vi "Example_OE1022 Sample.vi"() -> ()   [LabVIEW 2011]
uses:
  <vilib>/Utility/file.llb/Write To Spreadsheet File (DBL).vi
panel:
  out "输出数组":sgl[](array[numeric])
  out "diff_value":i32
  in  "Buffer":u16(ring) items=["R", "X", "Y", "Theta", "Rh1", "Xh1", "Yh1", "Theta h1", "Rh2", "Xh2", "Yh2", "Theta h2", "Noise", "A1", "A2", "A3", "A4", "E1", "E2", "E3", "E4", "Freq"]
  in  "Channel":i32(ring)=1 items=["1"=1, "2"=2, "3"=3, "4"=4]
  out "point":i32
  out "dis_flag":i32
  out "now_point":i32
  in  "Save Path":path=path "C:/Users/Joean/Desktop/123.xls"
  out "Output":sgl[](array[numeric])
  out "chart":sgl[](graph)
  in  "stop":bool
  in  "save":bool
  out "now_point":string
  out "Read Buffer":string
  in  "command":string
  in  "Remote Mode":u16(ring)=1 items=["USB", "RS232", "GPIB", "Ethernet"]
  in  "VISA resource name":refnum<visa-resource-name>
  in  "control_state":T1(ring)
  in  "drive_control":T2(ring)
  # "Tel          :   +86-020-84133345\nWebsite  :   www.ssi-instrument.com\nE-mail     :   support@si-instrument.com"
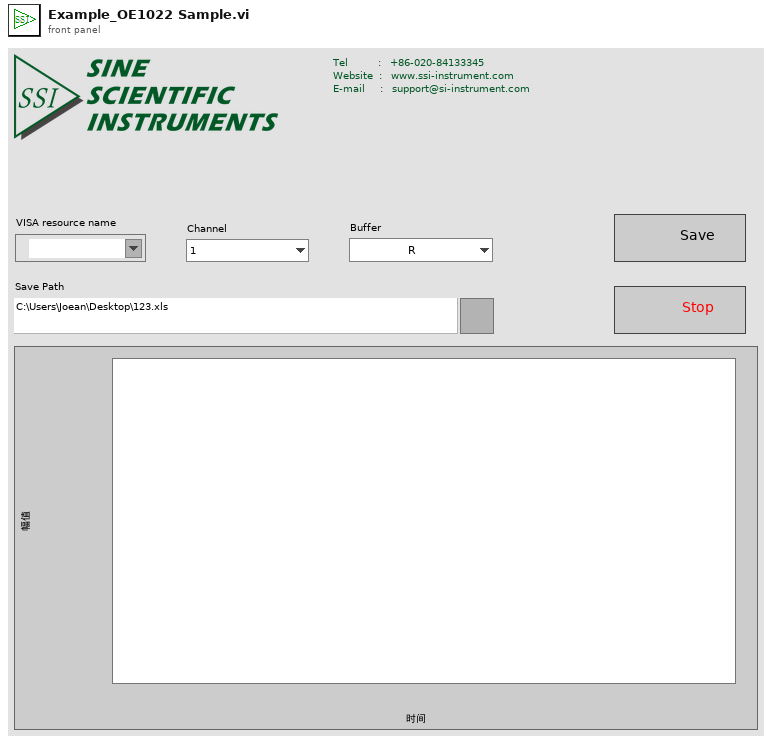
[diagram p1: front panel]
types:
  T1 = enum16{"connect", "initial", "idle", "set_channel", "sample", "save", "stop"}
  T2 = enum16{"idle", "initial", "write_cmd", "get_point", "read_data", "close"}
  T3 = enum16{"connect", "initial", "idle", "set_channel", "sample", "save", "stop", "close"}
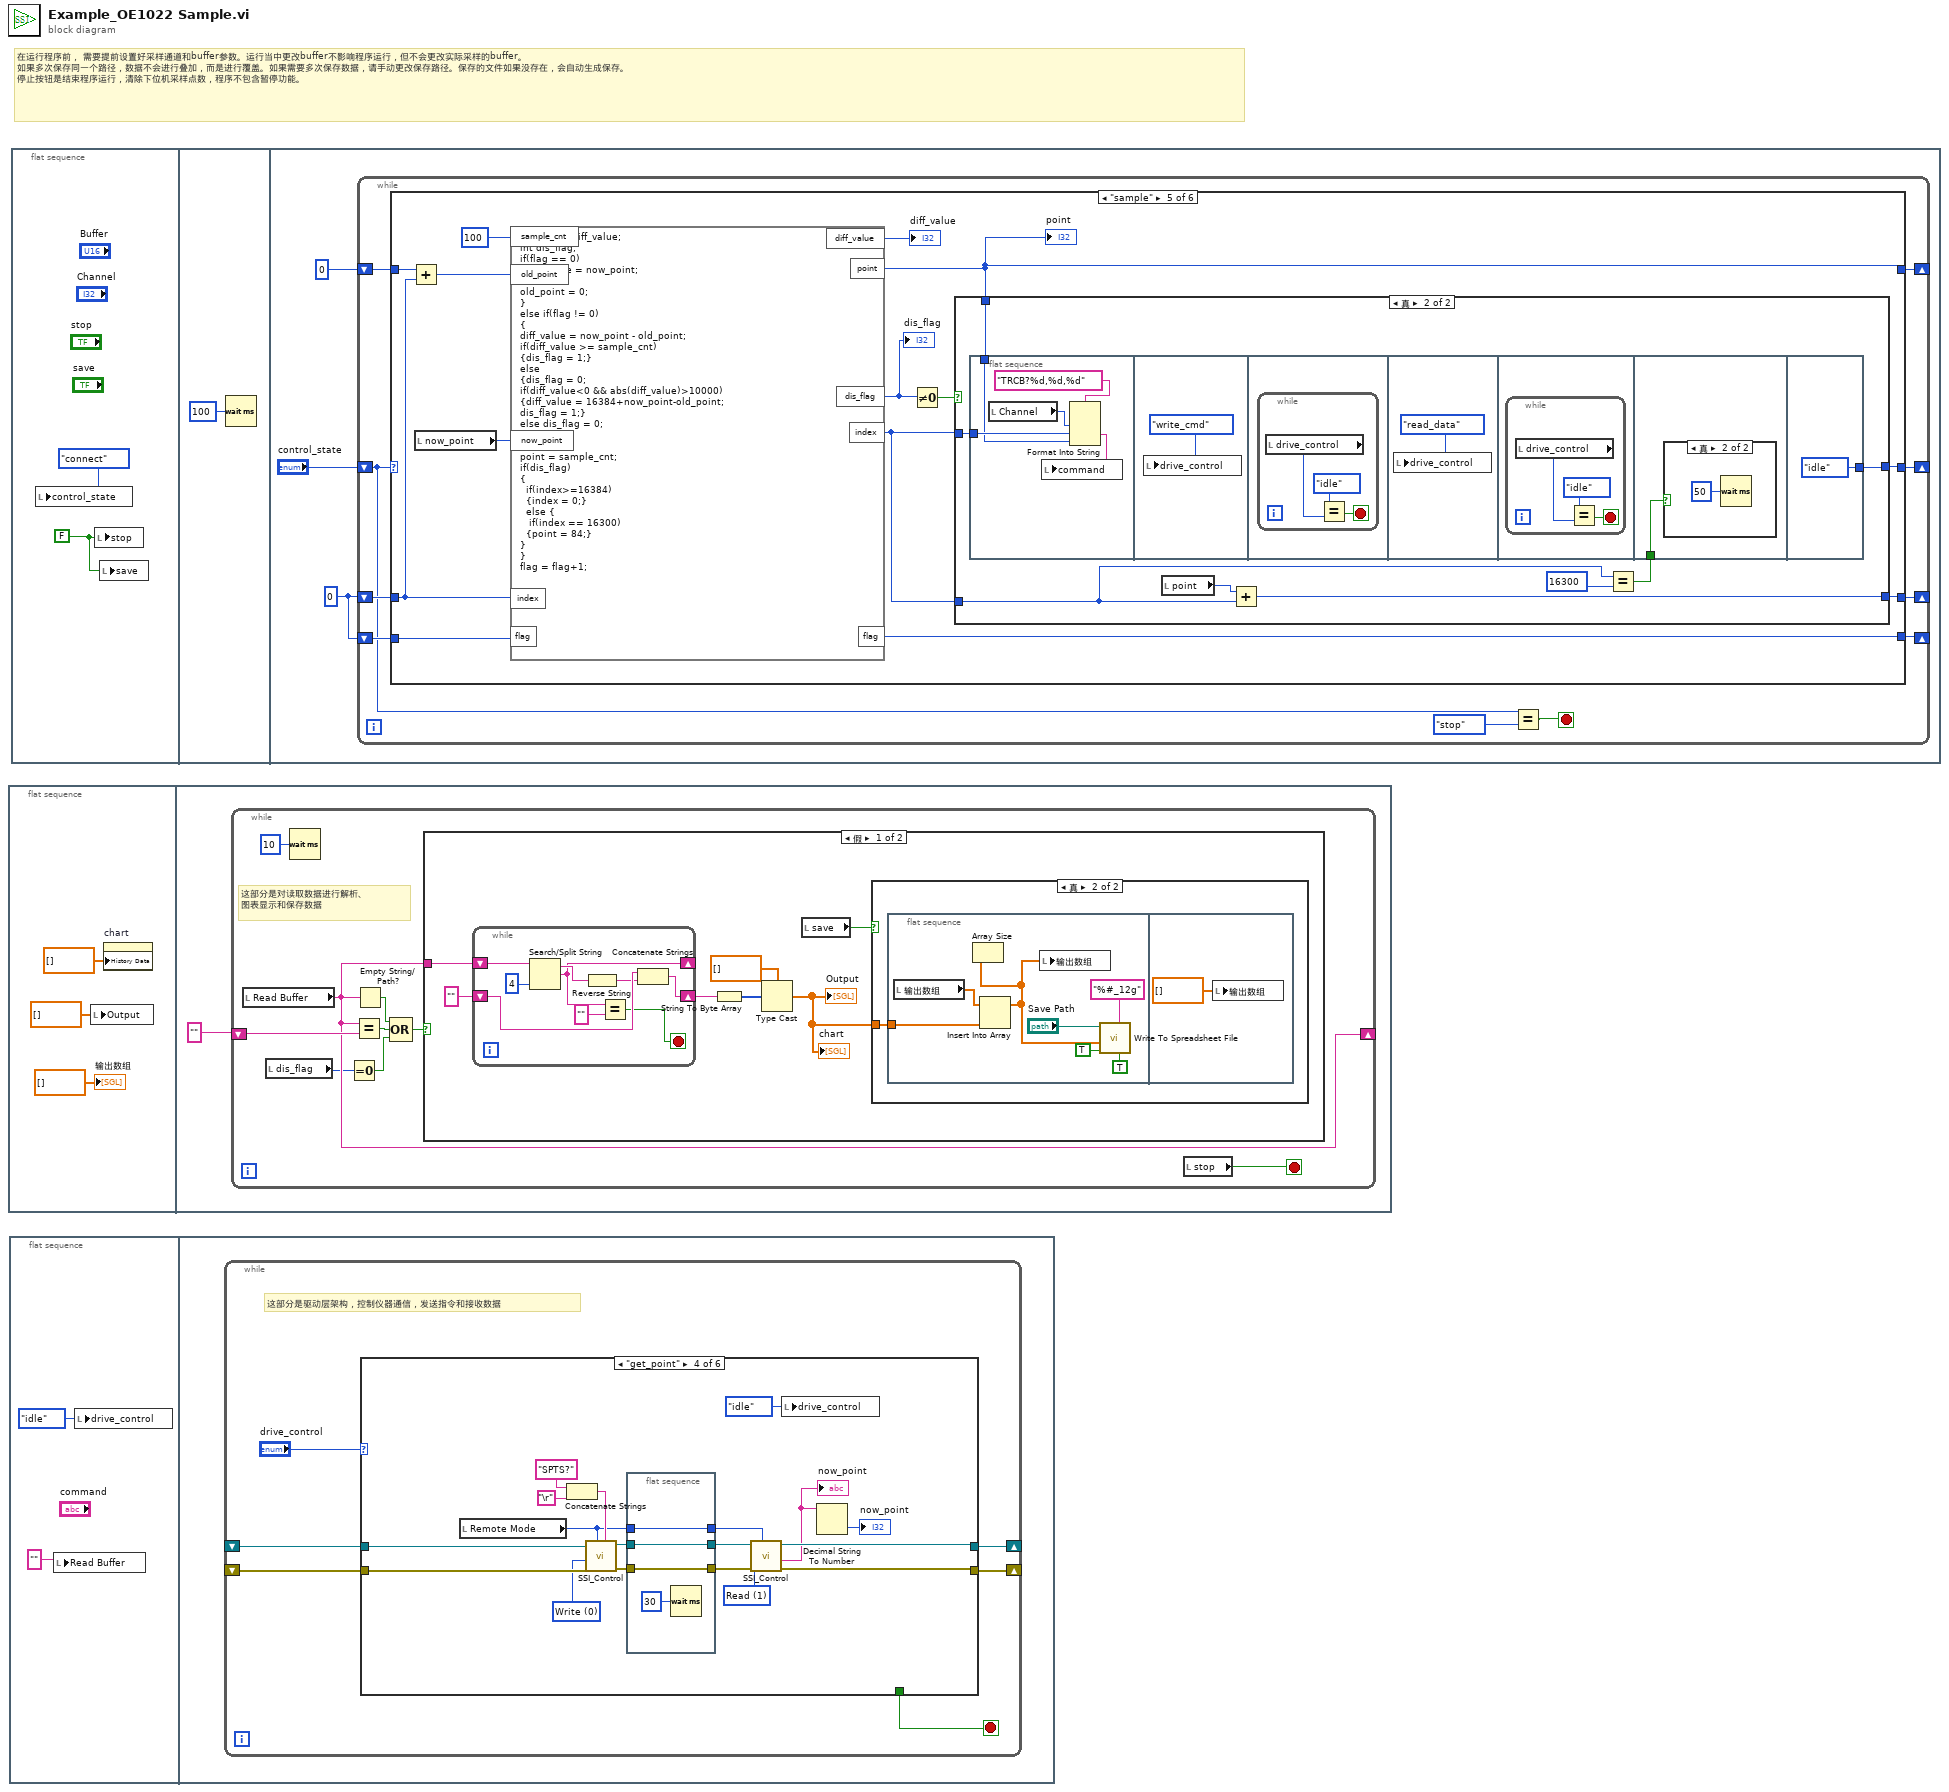
[diagram p0: block diagram]
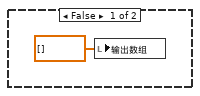
[diagram p2: hidden frame]
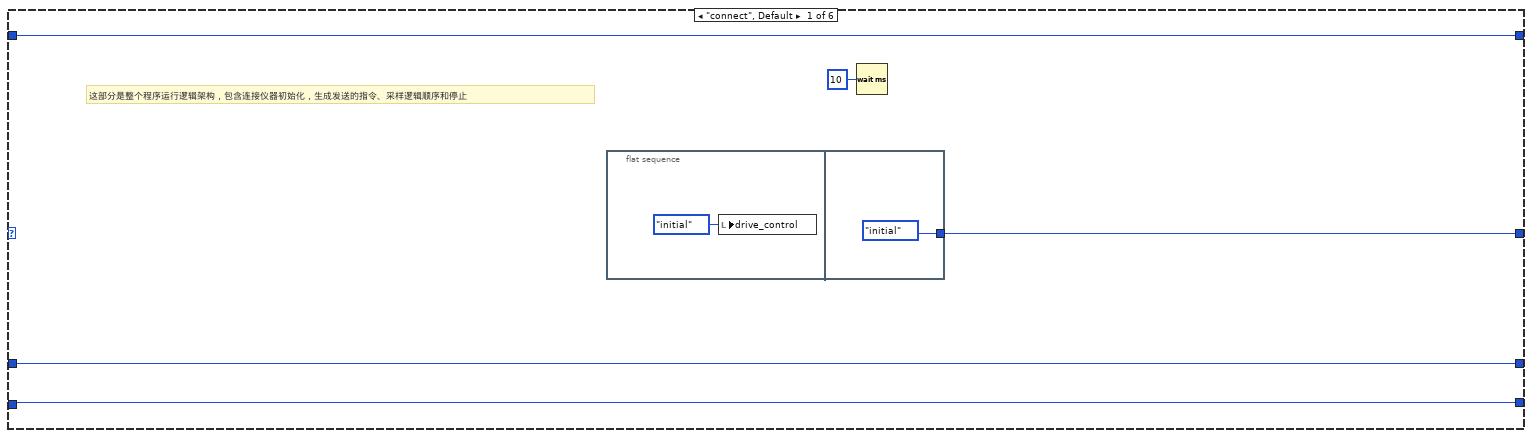
[diagram p4: hidden frame]
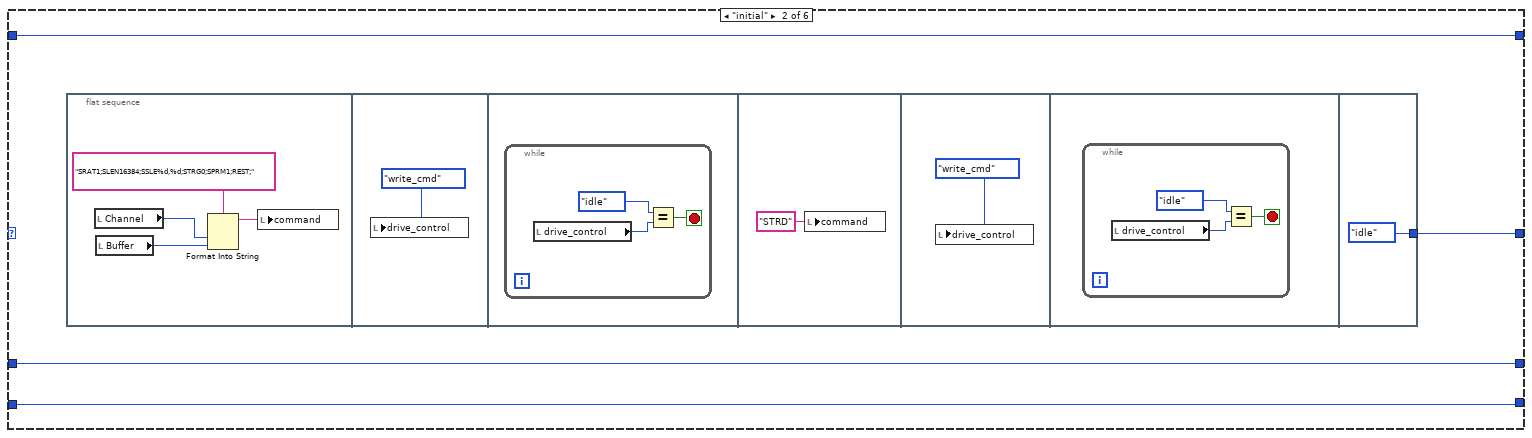
[diagram p5: hidden frame]
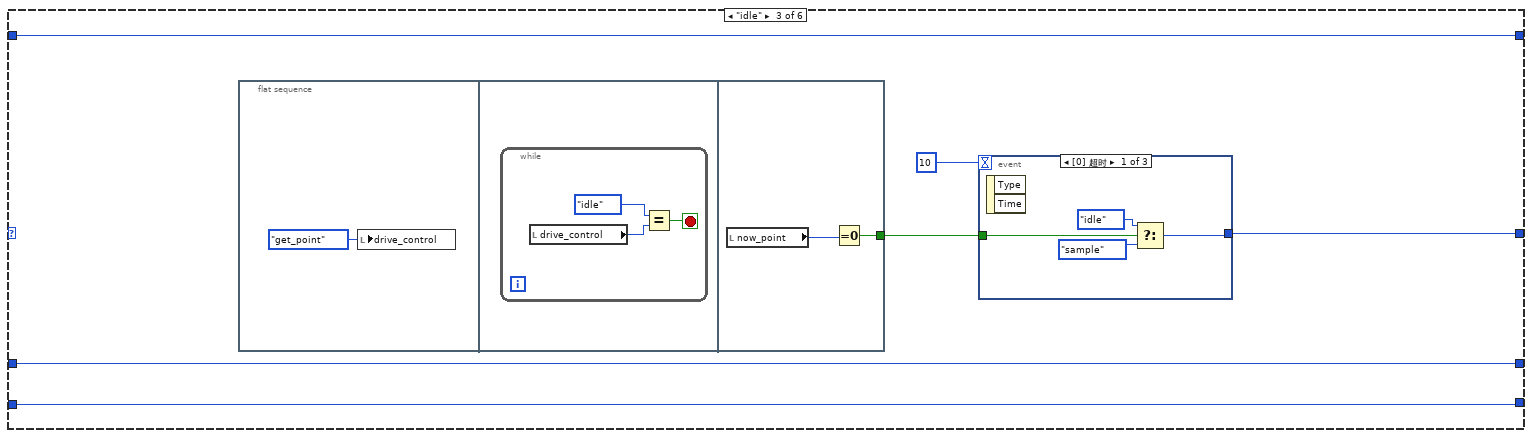
[diagram p6: hidden frame]
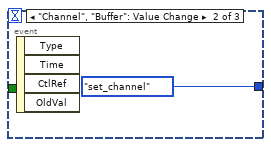
[diagram p7: hidden frame]
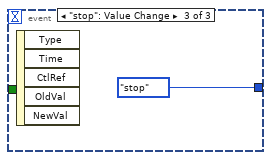
[diagram p8: hidden frame]
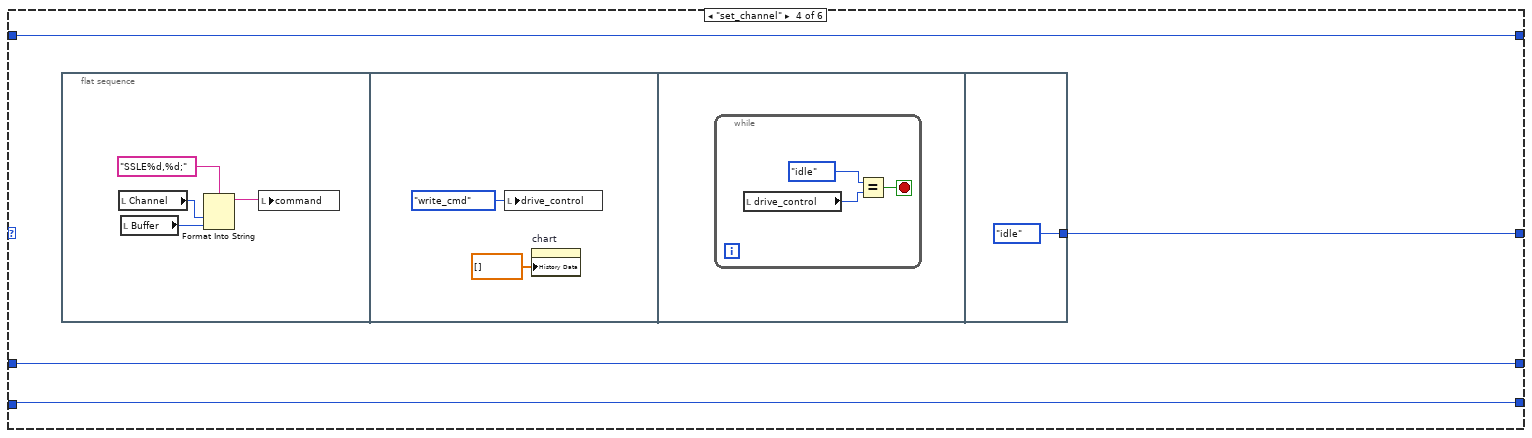
[diagram p9: hidden frame]
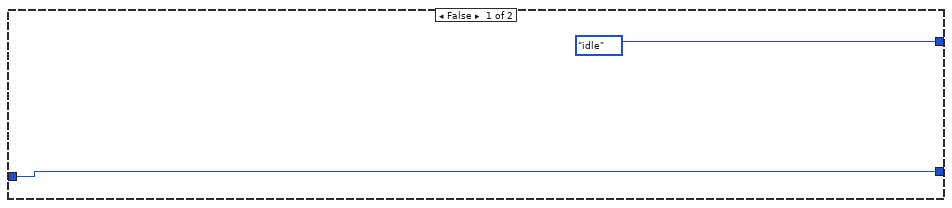
[diagram p10: hidden frame]
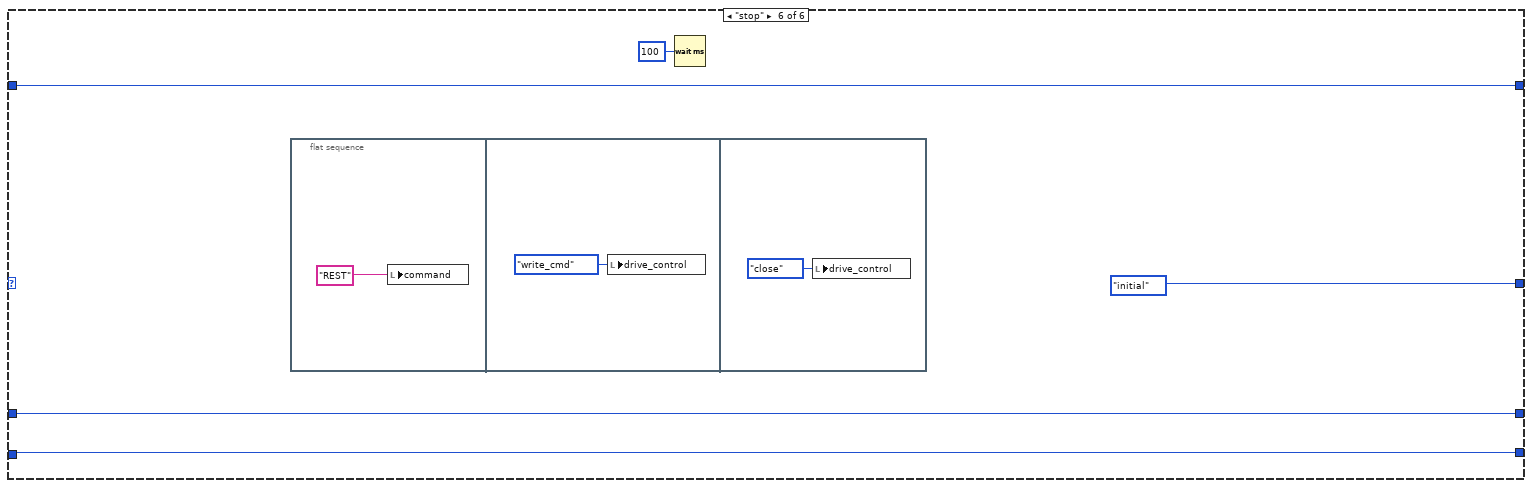
[diagram p12: hidden frame]
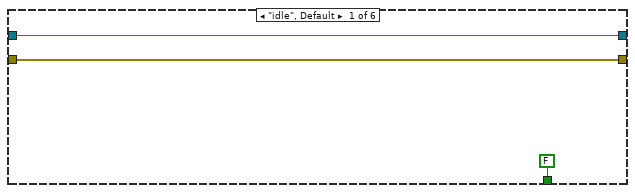
[diagram p13: hidden frame]
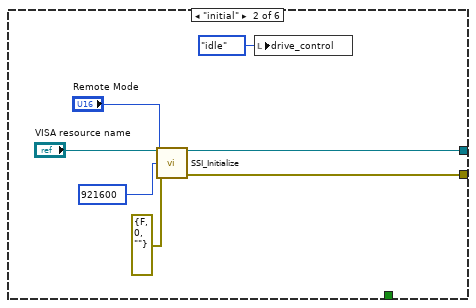
[diagram p14: hidden frame]
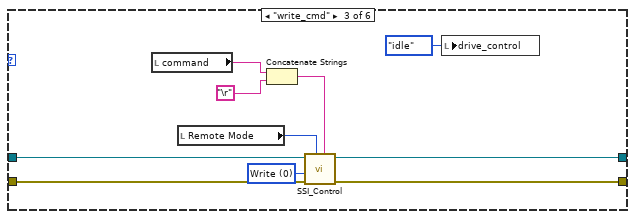
[diagram p15: hidden frame]
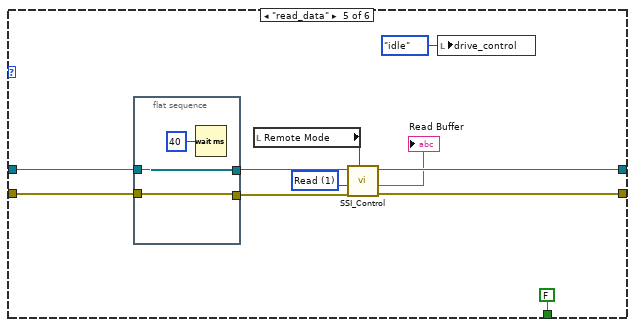
[diagram p16: hidden frame]
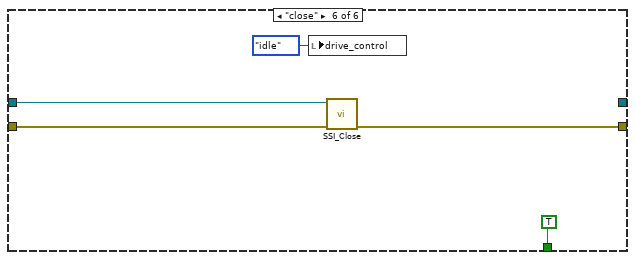
[diagram p17: hidden frame]
diagram:
  # "在运行程序前， 需要提前设置好采样通道和buffer参数。运行当中更改buffer不影响程序运行，但不会更改实际采样的buffer。\n如果多次保存同一个路径，数据不会进行叠加，而是进行覆盖。如果需要多次保存数据，请手动更改保存路径。保存的文件如果没存在，会自动生成保存。\n停止按钮是结束程序运行，清除下位机采样点数，程序不包含暂停功能。"
  n1 = flat-sequence {
    frame #0 {
      n2 = local write "Output"(sgl[] [] ("Output")) -> ()
      n3 = property on="chart" class="WFChart (严格)"("History Data"=sgl[] [] ("历史数据")) -> ()  [unwired: 2 in, 2 out]
      "输出数组" <- sgl[] [] ("输出数组")
    }
    frame #1 {
      n4 = while {
        shift-right: [w9] -> _
        shift-left: "" -> [w10]
        stop <- w12 stop-if-true
        # "这部分是对读取数据进行解析、\n图表显示和保存数据"
        n5 = local read "Read Buffer"() -> (w9:string)
        n6 = local read "dis_flag"() -> (w7:i32)
        n7 = Wait (ms)(milliseconds to wait=u32 10 ("等待时间（毫秒）")) -> ()  [unwired: 1 out]
        n8 = Equal To 0?(x=w7) -> (x = 0?=w6:bool)
        n9 = Equal?(x=w9, y=w10) -> (x = y?=w11:bool)
        n10 = Empty String/Path?(string/path=w9) -> (empty?=w8:bool)
        n11 = Compound Arithmetic op=OR(w8, w11, w6) -> (w5:bool)
        n12 = case shown="假" w5 {
          tunnel: w9 -> [w20 _]
          frame False {
            n13 = while {
              shift-right: [w33] -> _
              shift-left: w20 -> [w37]
              shift-right: [w34] -> w16
              shift-left: "" -> [w36]
              stop <- w31 stop-if-true
              n14 = Search/Split String(string=w37, offset (0)=4 ("偏移量(0)")) -> (substring before match=w38:string, match + rest of string=w33:string)  [unwired: 1 in, 1 out]
              n15 = Reverse String(1:w38) -> (0:w35:string)
              n16 = Equal?(x=w33, y="") -> (x = y?=w31:bool)
              n17 = Concatenate Strings(w36, w35) -> (w34:string)
            }
            n18 = String To Byte Array(string=w16) -> (unsigned byte array=w19:u8[])
            n19 = Type Cast(type=sgl[] [], x=w19) -> (*(type *) &x=w14:sgl[])
            "Output" <- w14
            "chart" <- w14
            n20 = local read "save"() -> (w15:bool)
            n21 = case shown="真" w15 {
              tunnel: w14 -> [_ w22]
              frame False {
                n22 = local write "输出数组"(sgl[] [] ("输出数组")) -> ()
              }
              frame True {
                n23 = flat-sequence {
                  tunnel: w22 -> [w25]
                  frame #0 {
                    n24 = local read "输出数组"() -> (w24:sgl[])
                    n25 = Insert Into Array(array=w24, new element=w25) -> (w23:sgl[])  [unwired: 1 in]
                    n26 = Array Size(array=w23) -> ()  [unwired: 1 out]
                    n27 = local write "输出数组"(w23) -> ()
                    n28 = call-poly <vilib>:"Write To Spreadsheet File.vi"("transpose? (no:F)"=TRUE, "format (%.3f)"="%#_12g", "append to file? (new file:F)"=TRUE, "1D data"=w23, "file path (dialog if empty)"="Save Path") -> ()  [unwired: 3 in, 1 out]
                  }
                  frame #1 {
                    n29 = local write "输出数组"(sgl[] [] ("输出数组")) -> ()
                  }
                }
              }
            }
          }
          frame True {
          }
        }
        n30 = local read "stop"() -> (w12:bool)
      }
    }
  }
  n31 = flat-sequence {
    frame #0 {
      n32 = local write "Read Buffer"("") -> ()
      n33 = local write "drive_control"(T2."idle" ("drive_control")) -> ()
    }
    frame #1 {
      n34 = while {
        shift-right: [w43] -> _
        shift-left: _ -> [w45]
        shift-right: [w44] -> _
        shift-left: _ -> [w46]
        stop <- w42 stop-if-true
        # "这部分是驱动层架构，控制仪器通信，发送指令和接收数据"
        n35 = case shown="\"get_point\"" "drive_control" {
          tunnel: [w50 w53 w65 w82 w99 _] -> w43
          tunnel: [w49 w52 w64 w81 w100 w108] -> w44
          tunnel: w45 -> [w50 _ w67 w85 w98 w105]
          tunnel: w46 -> [w49 _ w66 w84 w97 w104]
          tunnel: [FALSE _ _ _ FALSE TRUE] -> w42
          frame "idle", Default {
          }
          frame "initial" {
            n36 = call "SSI_Initialize.vi"("VISA resource name"="VISA resource name", "Remote Mode"="Remote Mode", "baud rate (921600)"=u32 921600, "error in (no error)"=errorcluster {"status"=FALSE, "code"=0, "source"=""}) -> ("VISA resource name out"=w53:refnum<visa-resource-name>, "error out"=w52:errorcluster)  [unwired: 9 in, 1 out]
            n37 = local write "drive_control"(T2."idle" ("drive_control")) -> ()
          }
          frame "write_cmd" {
            w63 = u16 0 items=["Write", "Read"] ("Control")
            n38 = local read "command"() -> (w59:string)
            n39 = local read "Remote Mode"() -> (w62:u16)
            n40 = Concatenate Strings(w59, "\r") -> (w60:string)
            n41 = call "SSI_Control.vi"("Write Buffer"=w60, "Remote Mode"=w62, "Error in (no error)"=w66, "Control"=w63, "VISA resource name"=w67) -> ("Error out"=w64:errorcluster, "VISA resource  out"=w65:refnum<visa-resource-name>)  [unwired: 3 in, 2 out]
            n42 = local write "drive_control"(T2."idle" ("drive_control")) -> ()
          }
          frame "get_point" {
            w76 = u16 1 items=["Write", "Read"] ("Control")
            w71 = u16 0 items=["Write", "Read"] ("Control")
            n43 = local read "Remote Mode"() -> (w70:u16)
            n44 = Concatenate Strings("SPTS?", "\r") -> (w80:string)
            n45 = call "SSI_Control.vi"("Write Buffer"=w80, "Remote Mode"=w70, "Error in (no error)"=w84, "Control"=w71, "VISA resource name"=w85) -> ("Error out"=w73:errorcluster, "VISA resource  out"=w72:refnum<visa-resource-name>)  [unwired: 3 in, 2 out]
            n46 = flat-sequence {
              tunnel: w72 -> [w89]
              tunnel: [w89] -> w75
              tunnel: w73 -> [w88]
              tunnel: [w88] -> w74
              tunnel: w70 -> [w86]
              tunnel: [w86] -> w77
              frame #0 {
                n47 = Wait (ms)(milliseconds to wait=u32 30 ("等待时间（毫秒）")) -> ()  [unwired: 1 out]
              }
            }
            n48 = call "SSI_Control.vi"("Remote Mode"=w77, "Error in (no error)"=w74, "Control"=w76, "VISA resource name"=w75) -> ("Error out"=w81:errorcluster, "Read Buffer"=w69:string, "VISA resource  out"=w82:refnum<visa-resource-name>)  [unwired: 4 in, 1 out]
            "now_point" <- w69
            n49 = local write "drive_control"(T2."idle" ("drive_control")) -> ()
            n50 = Decimal String To Number(string=w69) -> (number=→"now_point":i32)  [unwired: 2 in, 1 out]
          }
          frame "read_data" {
            w92 = u16 1 items=["Write", "Read"] ("Control")
            n51 = flat-sequence {
              tunnel: [w103] -> w90
              tunnel: w98 -> [w103]
              tunnel: [w102] -> w91
              tunnel: w97 -> [w102]
              frame #0 {
                n52 = Wait (ms)(milliseconds to wait=u32 40 ("等待时间（毫秒）")) -> ()  [unwired: 1 out]
              }
            }
            n53 = local read "Remote Mode"() -> (w93:u16)
            n54 = call "SSI_Control.vi"("Remote Mode"=w93, "Error in (no error)"=w91, "Control"=w92, "VISA resource name"=w90) -> ("Error out"=w100:errorcluster, "Read Buffer"=→"Read Buffer":string, "VISA resource  out"=w99:refnum<visa-resource-name>)  [unwired: 4 in, 1 out]
            n55 = local write "drive_control"(T2."idle" ("drive_control")) -> ()
          }
          frame "close" {
            n56 = local write "drive_control"(T2."idle" ("drive_control")) -> ()
            n57 = call "SSI_Close.vi"("Error in (no error)"=w104, "VISA resource name"=w105) -> ("Error out"=w108:errorcluster)  [unwired: 5 in]
          }
        }
      }
    }
  }
  n58 = flat-sequence {
    frame #0 {
      w110 = FALSE ("停止")
      n59 = local write "control_state"(T3."connect" ("control_state")) -> ()
      n60 = local write "stop"(w110) -> ()
      n61 = local write "save"(w110) -> ()
    }
    frame #1 {
      n62 = Wait (ms)(milliseconds to wait=u32 100 ("等待时间（毫秒）")) -> ()  [unwired: 1 out]
    }
    frame #2 {
      w112 = 0
      n63 = while {
        shift-right: [w117] -> _
        shift-left: "control_state" -> [w115]
        shift-right: [w122] -> _
        shift-left: 0 -> [w124]
        shift-right: [w121] -> _
        shift-left: w112 -> [w123]
        shift-right: [w120] -> _
        shift-left: w112 -> [w119]
        stop <- w118 stop-if-true
        n64 = case shown="\"sample\"" w115 {
          tunnel: [w126 w132 w154 w168 w186 T3."initial" ("control_state")] -> w117
          tunnel: w124 -> [w129 w134 w150 w171 w189 w226]
          tunnel: w123 -> [w128 w135 w152 w170 w187 w225]
          tunnel: w119 -> [w127 w133 w151 w169 w195 w224]
          tunnel: [w127 w133 w151 w169 w194 w224] -> w120
          tunnel: [w129 w134 w150 w171 w182 w226] -> w122
          tunnel: [w128 w135 w152 w170 w184 w225] -> w121
          frame "connect", Default {
            # "这部分是整个程序运行逻辑架构，包含连接仪器初始化，生成发送的指令、采样逻辑顺序和停止"
            n65 = flat-sequence {
              tunnel: [T3."initial" ("control_state")] -> w126
              frame #0 {
                n66 = local write "drive_control"(T2."initial" ("drive_control")) -> ()
              }
              frame #1 {
              }
            }
            n67 = Wait (ms)(milliseconds to wait=u32 10 ("等待时间（毫秒）")) -> ()  [unwired: 1 out]
          }
          frame "initial" {
            n68 = flat-sequence {
              tunnel: [T3."idle" ("control_state")] -> w132
              frame #0 {
                n69 = local read "Channel"() -> (w136:i32)
                n70 = local read "Buffer"() -> (w137:u16)
                n71 = Format Into String(format string="SRAT1;SLEN16384;SSLE%d,%d;STRG0;SPRM1;REST;", w136, w137) -> (resulting string=w138:string)  [unwired: 2 in, 1 out]
                n72 = local write "command"(w138) -> ()
              }
              frame #1 {
                n73 = local write "drive_control"(T2."write_cmd" ("drive_control")) -> ()
              }
              frame #2 {
                n74 = while {
                  stop <- w141 stop-if-true
                  n75 = local read "drive_control"() -> (w142:T2)
                  n76 = Equal?(x=T2."idle" ("drive_control"), y=w142) -> (x = y?=w141:bool)
                }
              }
              frame #3 {
                n77 = local write "command"("STRD" ("command")) -> ()
              }
              frame #4 {
                n78 = local write "drive_control"(T2."write_cmd" ("drive_control")) -> ()
              }
              frame #5 {
                n79 = while {
                  stop <- w146 stop-if-true
                  n80 = local read "drive_control"() -> (w147:T2)
                  n81 = Equal?(x=T2."idle" ("drive_control"), y=w147) -> (x = y?=w146:bool)
                }
              }
              frame #6 {
              }
            }
          }
          frame "idle" {
            n82 = flat-sequence {
              tunnel: [w161] -> w153
              frame #0 {
                n83 = local write "drive_control"(T2."get_point" ("drive_control")) -> ()
              }
              frame #1 {
                n84 = while {
                  stop <- w157 stop-if-true
                  n85 = local read "drive_control"() -> (w158:T2)
                  n86 = Equal?(x=T2."idle" ("drive_control"), y=w158) -> (x = y?=w157:bool)
                }
              }
              frame #2 {
                n87 = local read "now_point"() -> (w160:i32)
                n88 = Equal To 0?(x=w160) -> (x = 0?=w161:bool)
              }
            }
            n89 = event shown="[0] 超时" {
              selector: _ -> [_ _ _]
              dyn-events: _ -> [_ _ _]
              timeout: 10 -> [_ _ _]
              tunnel: [w164 T3."set_channel" ("f") T3."stop" ("f")] -> w154
              tunnel: w153 -> [w165 _ _]
              event Timeout {
                n90 = event-data() -> ()  [unwired: 1 in, 2 out]
                n91 = Select(t=T3."idle" ("control_state"), s=w165, f=T3."sample") -> (s? t:f=w164:T3)
              }
              event "Channel", "Buffer": Value Change {
                n92 = event-data() -> ()  [unwired: 1 in, 4 out]
              }
              event "stop": Value Change {
                n93 = event-data() -> ()  [unwired: 1 in, 5 out]
              }
            }
          }
          frame "set_channel" {
            n94 = flat-sequence {
              tunnel: [T3."idle" ("control_state")] -> w168
              frame #0 {
                n95 = local read "Channel"() -> (w173:i32)
                n96 = local read "Buffer"() -> (w172:u16)
                n97 = Format Into String(format string="SSLE%d,%d;" ("格式字符串"), w173, w172) -> (resulting string=w175:string)  [unwired: 2 in, 1 out]
                n98 = local write "command"(w175) -> ()
              }
              frame #1 {
                n99 = local write "drive_control"(T2."write_cmd" ("drive_control")) -> ()
                n100 = property on="chart" class="WFChart (严格)"("History Data"=sgl[] [] ("历史数据")) -> ()  [unwired: 2 in, 2 out]
              }
              frame #2 {
                n101 = while {
                  stop <- w178 stop-if-true
                  n102 = local read "drive_control"() -> (w179:T2)
                  n103 = Equal?(x=T2."idle" ("drive_control"), y=w179) -> (x = y?=w178:bool)
                }
              }
              frame #3 {
              }
            }
          }
          frame "sample" {
            n104 = Add(x=w189, y=w187) -> (x+y=w188:i32)
            n105 = local read "now_point"() -> (w192:i32)
            n106 = formula code="int point,x,diff_value;\nint dis_flag;\nif(flag == 0)\n{diff_value = now_point;\nindex = 0;\nold_point = 0;\n}\nelse if(flag != 0)\n{\ndiff_value = now_point - old_point;\nif(diff_value >= sample_cnt)\n{dis_flag = 1;}\nelse\n{dis_flag = 0;\nif(diff_value<0 && abs(diff_value)>10000)\n{diff_value = 16384+now_point-old_point;\ndis_flag = 1;}\nelse dis_flag = 0;\n}\n}\npoint = sample_cnt;\nif(dis_flag)\n{\n  if(index>=16384)\n  {index = 0;}\n  else {\n   if(index == 16300)\n  {point = 84;}\n}\n}\nflag = flag+1;"("index"=w187, "flag"=w195, "sample_cnt"=u32 100 ("输入变量"), "now_point"=w192, "old_point"=w188) -> ("point"=w182:i32, "index"=w185:i32, "flag"=w194:i32, "dis_flag"=w190:i32, "diff_value"=→"diff_value":i32)
            "dis_flag" <- w190
            "point" <- w182
            n107 = Not Equal To 0?(x=w190) -> (x != 0?=w191:bool)
            n108 = case shown="真" w191 {
              tunnel: w185 -> [_ w205]
              tunnel: w182 -> [_ w204]
              tunnel: [T3."idle" ("control_state") w198] -> w186
              tunnel: w185 -> [w196 w200]
              tunnel: [w196 w201] -> w184
              frame False {
              }
              frame True {
                n109 = flat-sequence {
                  tunnel: w205 -> [w209]
                  tunnel: w204 -> [w208]
                  tunnel: w199 -> [w219]
                  tunnel: [T3."idle" ("control_state")] -> w198
                  frame #0 {
                    n110 = local read "Channel"() -> (w206:i32)
                    n111 = Format Into String(format string="TRCB?%d,%d,%d", w206, w209, w208) -> (resulting string=w207:string)  [unwired: 2 in, 1 out]
                    n112 = local write "command"(w207) -> ()
                  }
                  frame #1 {
                    n113 = local write "drive_control"(T2."write_cmd" ("drive_control")) -> ()
                  }
                  frame #2 {
                    n114 = while {
                      stop <- w212 stop-if-true
                      n115 = local read "drive_control"() -> (w213:T2)
                      n116 = Equal?(x=T2."idle" ("drive_control"), y=w213) -> (x = y?=w212:bool)
                    }
                  }
                  frame #3 {
                    n117 = local write "drive_control"(T2."read_data" ("drive_control")) -> ()
                  }
                  frame #4 {
                    n118 = while {
                      stop <- w216 stop-if-true
                      n119 = local read "drive_control"() -> (w217:T2)
                      n120 = Equal?(x=T2."idle" ("drive_control"), y=w217) -> (x = y?=w216:bool)
                    }
                  }
                  frame #5 {
                    n121 = case shown="真" w219 {
                      frame False {
                      }
                      frame True {
                        n122 = Wait (ms)(milliseconds to wait=u32 50 ("等待时间（毫秒）")) -> ()  [unwired: 1 out]
                      }
                    }
                  }
                  frame #6 {
                  }
                }
                n123 = local read "point"() -> (w203:i32)
                n124 = Add(x=w203, y=w200) -> (x+y=w201:i32)
                n125 = Equal?(x=w200, y=16300) -> (x = y?=w199:bool)
              }
            }
          }
          frame "stop" {
            n126 = flat-sequence {
              frame #0 {
                n127 = local write "command"("REST") -> ()
              }
              frame #1 {
                n128 = local write "drive_control"(T2."write_cmd" ("drive_control")) -> ()
              }
              frame #2 {
                n129 = local write "drive_control"(T2."close" ("drive_control")) -> ()
              }
            }
            n130 = Wait (ms)(milliseconds to wait=u32 100 ("等待时间（毫秒）")) -> ()  [unwired: 1 out]
          }
        }
        n131 = Equal?(x=w115, y=T3."stop") -> (x = y?=w118:bool)
      }
    }
  }
